vi "View.vi"(8 "error in (no error)":errorcluster, 11 "Camera View in":refnum<class "Camera View.lvclass">) -> (0 "error out":errorcluster, 3 "Camera View out":refnum<class "Camera View.lvclass">)   [LabVIEW 2022 SP3, in "Camera View.lvclass"]
uses:
  Camera View.lvclass
  C:/XY Stage/iView/base view/base view.lvclass
  7f8fb19e-39f1-4a5d-adf9-baa751c50954.vi
  0434362a-7b1f-4b1a-b8b1-85615a5f48f8.vi
  Accessors/Read Camera Controller.lvclass.vi
  iView/base view/Accessors/Read Events.vi
  iView/base view/base view.lvclass
  Camera Controller/Camera Controller.lvclass
  Camera View.lvclass/Camera View.ctl
panel:
  out "Image Display":T1(plugin-control)
  out "Standard Varition":dbl
  out "Mean":dbl
  out "Max":dbl
  out "Min":dbl
  in  "Save Path":path
  in  "Save Image":bool
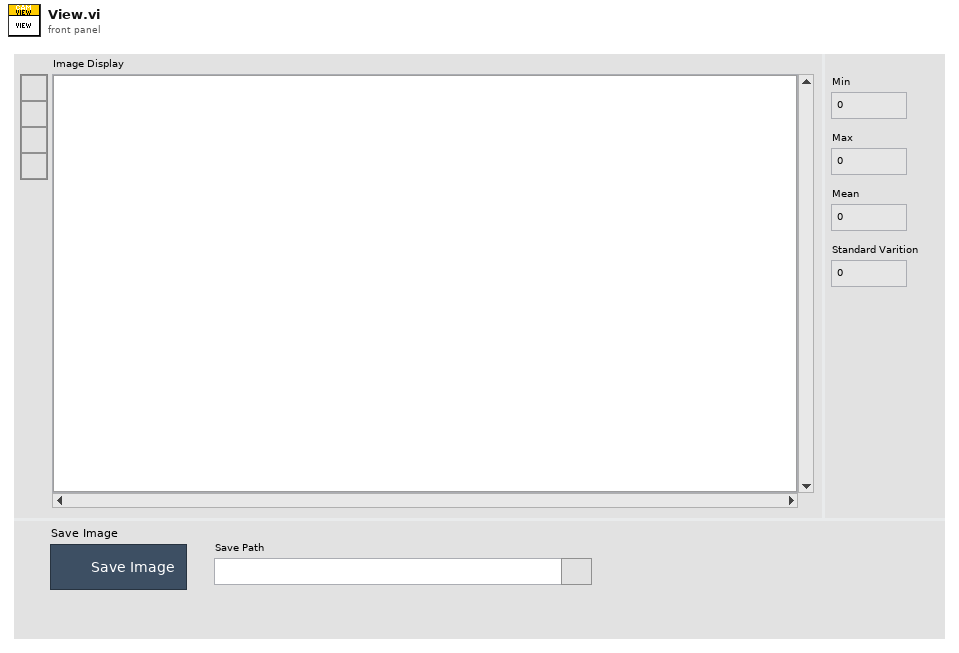
[diagram p1: front panel]
types:
  T1 = typedef "IMAQ Image.ctl" = refnum<image>
  T2 = typedef "base view.lvclass/Events.ctl" = cluster{"Open":refnum<user-event>, "Close":refnum<user-event>, "Hide":refnum<user-event>}
  T3 = cluster{"Event Registration Refnum":refnum<event-registration>, "Event Registration Refnum":refnum<event-registration>}
  T4 = cluster{"Event Registration Refnum":refnum<event-registration>, "Event Registration Refnum":refnum<event-registration>, "Event Registration Refnum":refnum<event-registration>}
  T5 = cluster{"Global Rectangle":i32[], "Contours":cluster{"Contour Type":u32, "ROI Type":u32, "Points":i32[]}[]}
  T6 = cluster{"Global Rectangle":bool[], "Contours":cluster{"Contour Type":bool, "ROI Type":bool, "Points":bool[]}[]}
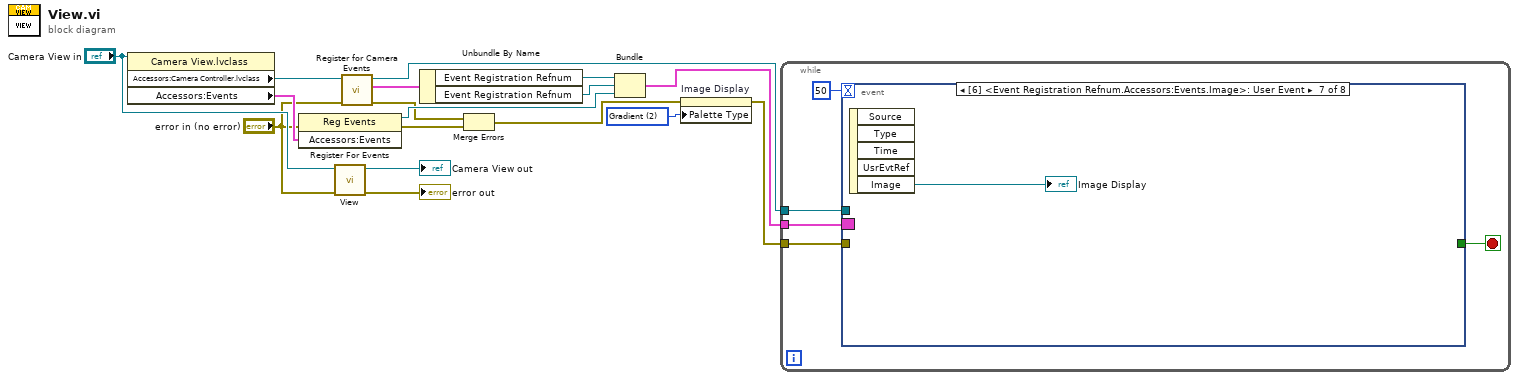
[diagram p0: block diagram]
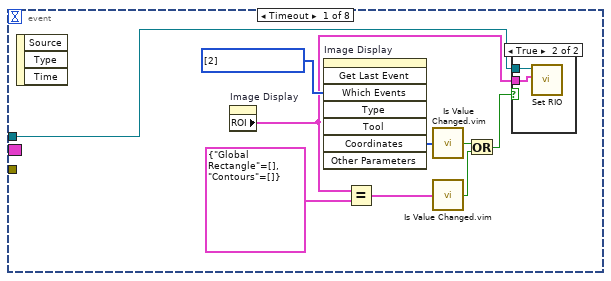
[diagram p2: hidden frame]
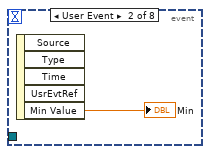
[diagram p4: hidden frame]
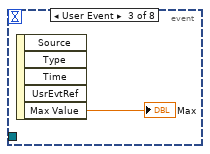
[diagram p5: hidden frame]
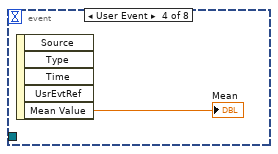
[diagram p6: hidden frame]
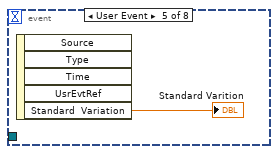
[diagram p7: hidden frame]
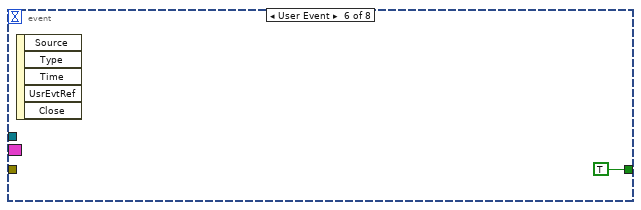
[diagram p8: hidden frame]
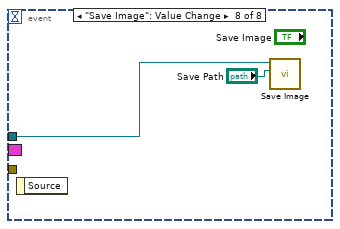
[diagram p9: hidden frame]
diagram:
  w6 = u32 2 items=["Grayscale", "Binary", "Gradient", "Rainbow", "Temperature", "User Defined", "Binary 16 Bit", "Gradient 16 Bit", "Rainbow 16 Bit", "Temperature 16 Bit", "User Defined 16 Bit"] ("Palette:Palette Type")
  n1 = property class="Camera View.lvclass"(reference="Camera View in") -> ("Accessors:Camera Controller.lvclass"=w9:refnum<class "Camera Controller.lvclass">, "Accessors:Events"=w8:T2)  [unwired: 1 in, 2 out]
  n2 = register-events(error in="error in (no error)", w8) -> (reference out=w11:refnum<event-registration>, error out=w3:errorcluster)  [unwired: 1 in]
  n3 = call-parent "View.vi"("error in (no error)"="error in (no error)", "base view in"="Camera View in") -> ("error out"=→"error out":errorcluster, "base view out"=→"Camera View out":refnum<class "Camera View.lvclass">)  [unwired: 8 in]
  n4 = call-dynamic "Register for Camera Events.vi"("error in (no error)"="error in (no error)", "Camera Controller in"=w9) -> ("error out"=w4:errorcluster, "output cluster"=w14:T3, "Camera Controller out"=w7:refnum<class "Camera Controller.lvclass">)  [unwired: 7 in]
  n5 = Unbundle By Name(w14) -> ("Event Registration Refnum"=w13:refnum<event-registration>, "Event Registration Refnum"=w12:refnum<event-registration>)
  n6 = Merge Errors(w4, w3) -> (w2:errorcluster)
  n7 = Bundle("Event Registration Refnum"=w13, "Event Registration Refnum"=w12, "Event Registration Refnum"=w11) -> (w10:T4)  [unwired: 1 in]
  n8 = property on="Image Display" class="ImageControl"(error in=w2, "Palette Type"=w6) -> (error out=w1:errorcluster)  [unwired: 1 in, 1 out]
  n9 = while {
    tunnel: w10 -> [w22]
    tunnel: w7 -> [w20]
    tunnel: w1 -> [w18]
    stop <- w21 stop-if-true
    n10 = event shown="[6] <Event Registration Refnum.Accessors:Events.Image>: User Event" {
      selector: w22 -> [_ _ _ _ _ _ _ _]
      dyn-events: _ -> [_ _ _ _ _ _ _ _]
      timeout: 50 -> [_ _ _ _ _ _ _ _]
      tunnel: [_ _ _ _ _ TRUE _ _] -> w21
      tunnel: w20 -> [w24 _ _ _ _ _ _ w41]
      tunnel: w18 -> [_ _ _ _ _ _ _ _]
      event Timeout {
        w29 = i32[] [2] items=["No Event"=0, "Click Event"=1, "Draw Event"=2, "Size Event"=4, "Scroll Event"=5, "Double Click Event"=8] ("Which Events")
        n11 = event-data() -> ()  [unwired: 1 in, 3 out]
        n12 = property on="Image Display" class="ImageControl"() -> ("ROI"=w23:T5)  [unwired: 2 in, 2 out]
        n13 = invoke on="Image Display" class="ImageControl" method="Get Last Event"("Which Events"=w29) -> ("Coordinates"=w28:i32[])  [unwired: 7 in, 7 out]
        n14 = Equal?(x=w23, y=T5 {"Global Rectangle"=[], "Contours"=[]}) -> (x = y?=w30:T6)
        n15 = call "Is Value Changed.vim"("value"=w28) -> ("changed or first call?"=w27:bool)
        n16 = call "Is Value Changed.vim"("value"=w30) -> ("changed or first call?"=w26:bool)
        n17 = Or(x=w27, y=w26) -> (x .or. y?=w25:bool)
        n18 = case shown="True" w25 {
          tunnel: w24 -> [_ w33]
          tunnel: w23 -> [_ w32]
          frame False {
          }
          frame True {
            n19 = call-dynamic "Set RIO.vi"("ROI"=w32, "Camera Controller in"=w33) -> ()  [unwired: 8 in, 2 out]
          }
        }
      }
      event User Event {
        n20 = event-data() -> ("Min Value"=→"Min":dbl)  [unwired: 1 in, 4 out]
      }
      event User Event {
        n21 = event-data() -> ("Max Value"=→"Max":dbl)  [unwired: 1 in, 4 out]
      }
      event User Event {
        n22 = event-data() -> ("Mean Value"=→"Mean":sgl)  [unwired: 1 in, 4 out]
      }
      event User Event {
        n23 = event-data() -> ("Standard  Variation"=→"Standard Varition":sgl)  [unwired: 1 in, 4 out]
      }
      event User Event {
        n24 = event-data() -> ()  [unwired: 1 in, 5 out]
      }
      event User Event {
        n25 = event-data() -> ("Image"=→"Image Display":T1)  [unwired: 1 in, 4 out]
      }
      event "Save Image": Value Change {
        n26 = event-data() -> ()  [unwired: 1 in, 1 out]
        n27 = call-dynamic "Save Image.vi"("Path"="Save Path", "Camera Controller in"=w41) -> ()  [unwired: 8 in, 2 out]
      }
    }
  }
